vi "Images_Overlay_test.vi"() -> ()   [LabVIEW 2018]
uses:
  Common_Resources.lvlib
panel:
  out "error out":errorcluster
  out "Waveform Chart":dbl(graph)
  in  "Stop":bool
  in  "Image Display":T1(plugin-control)
  out "size(s)":i32[](array[numeric])
  in  "Overlay Object":path=path "D:/Users_Data/Dmitriy_T/Documents/Tracker/TestVI's/Overlay_Object.png"
  in  "Overlay Bgr":path=path "D:/Users_Data/Dmitriy_T/Documents/Tracker/TestVI's/Overlay_Bgr.png"
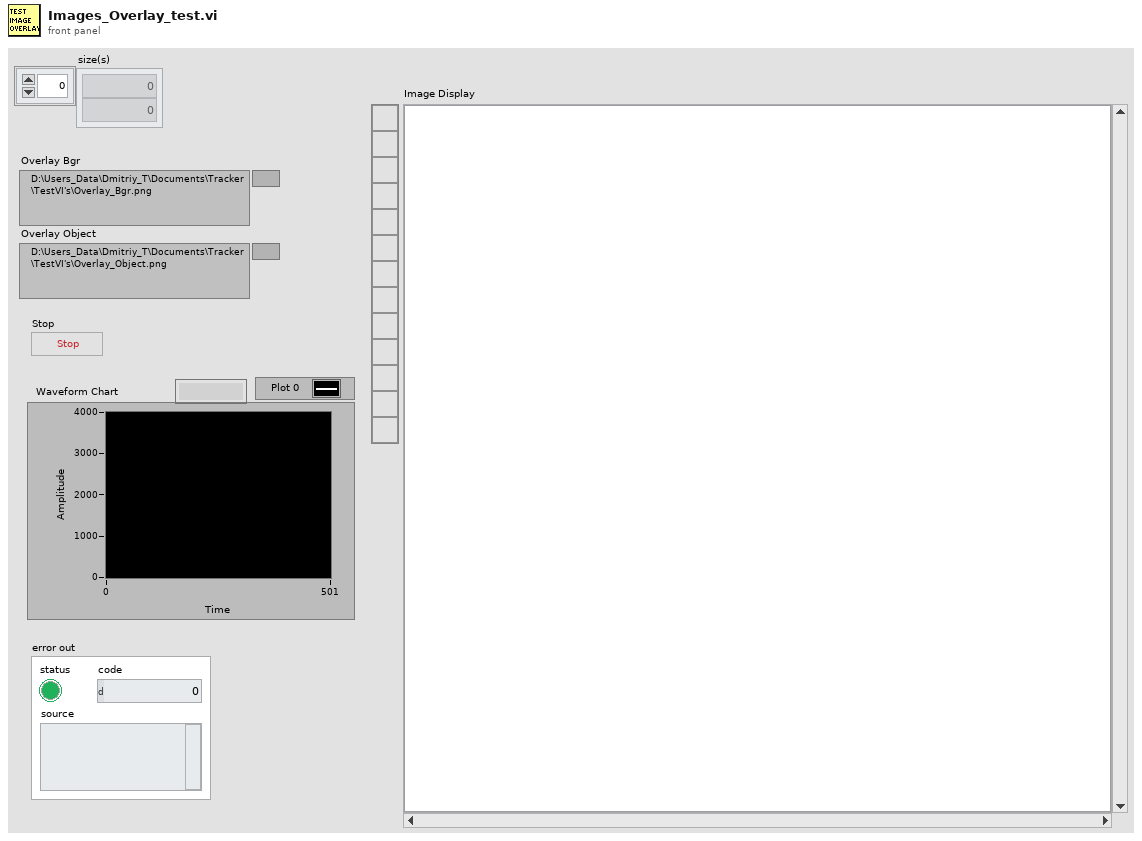
[diagram p1: front panel]
types:
  T1 = typedef "IMAQ Image.ctl" = refnum<image>
  T2 = typedef "Image Type" = u32
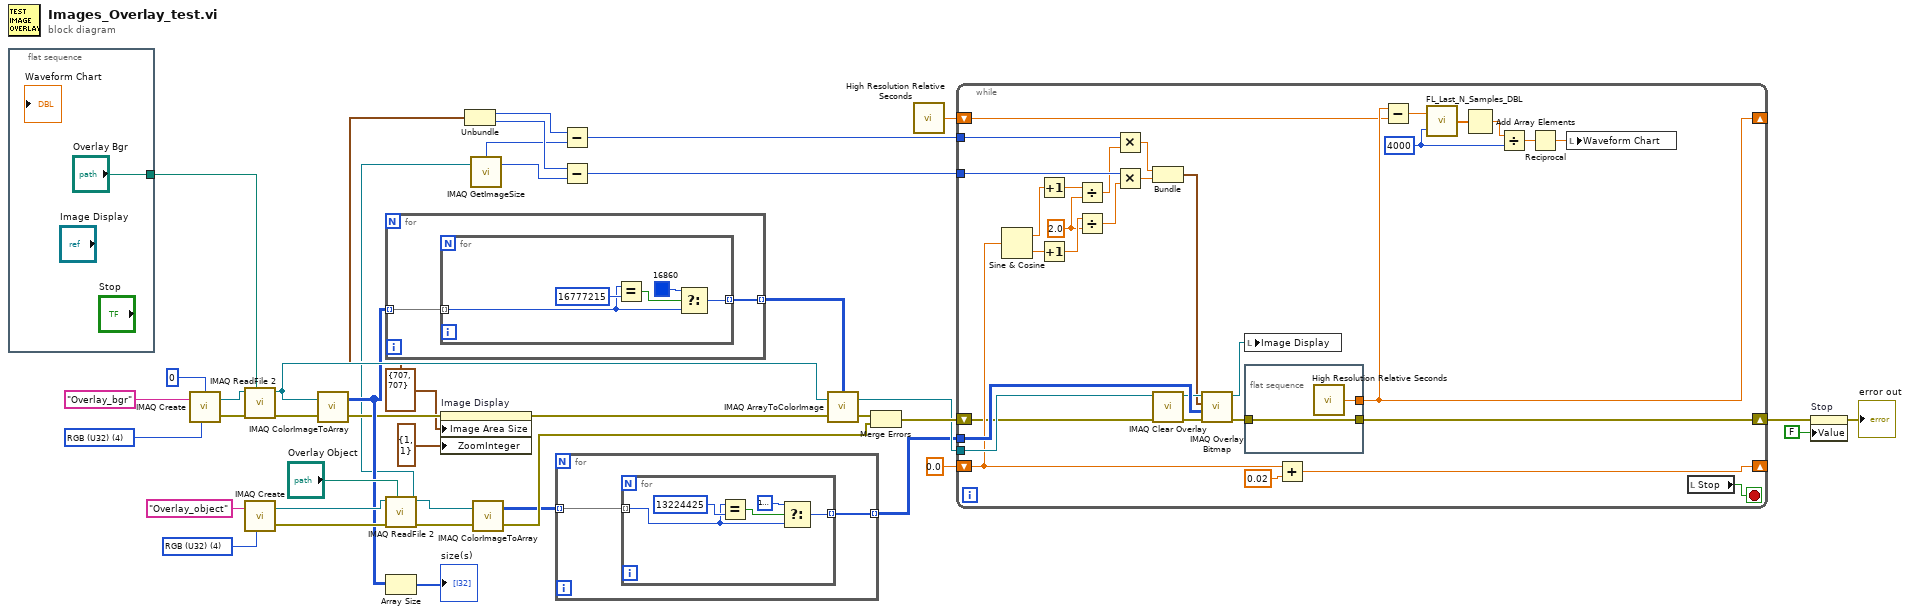
[diagram p0: block diagram]
diagram:
  w15 = cluster{"Width":u32, "Height":u32} {"Width"=707, "Height"=707} ("Image Area:Size:All Elements")
  w37 = T2 4 items=["Grayscale (U8)", "Grayscale (I16)", "Grayscale (SGL)", "Complex (CSG)", "RGB (U32)", "HSL (U32)", "RGB (U64)", "Grayscale (U16)"] ("Image Type")
  w38 = T2 4 items=["Grayscale (U8)", "Grayscale (I16)", "Grayscale (SGL)", "Complex (CSG)", "RGB (U32)", "HSL (U32)", "RGB (U64)", "Grayscale (U16)"] ("Image Type")
  n1 = flat-sequence {
    tunnel: ["Overlay Bgr"] -> w5
    frame #0 {
    }
  }
  n2 = call "IMAQ Create"("Border Size"=0, "Image Name"="Overlay_bgr", "Image Type"=w38) -> ("New Image"=w35:T1, "error out"=w34:errorcluster)  [unwired: 2 in]
  n3 = call "IMAQ ReadFile 2"("File Path"=w5, "error in (no error)"=w34, "Image"=w35) -> ("error out"=w26:errorcluster, "Image Out"=w23:T1)  [unwired: 4 in, 3 out]
  n4 = call "IMAQ Create"("Image Name"="Overlay_object", "Image Type"=w37) -> ("New Image"=w33:T1, "error out"=w32:errorcluster)  [unwired: 3 in]
  n5 = call "IMAQ ColorImageToArray"("Image"=w23, "error in (no error)"=w26) -> ("Image Pixels (U32)"=w22:u32[][], "error out"=w20:errorcluster)  [unwired: 2 in, 1 out]
  n6 = for {
    tunnel: w22 -> [w42] mode=indexing
    tunnel: [w41] -> w27 mode=indexing
    n7 = for {
      tunnel: w42 -> [w44] mode=indexing
      tunnel: [w46] -> w41 mode=indexing
      n8 = Equal?(x=w44, y=u32 16777215) -> (x = y?=w45:bool)
      n9 = Select(t=u32 16860, s=w45, f=w44) -> (s? t:f=w46:u32)
    }
  }
  n10 = call "IMAQ ReadFile 2"("File Path"="Overlay Object", "error in (no error)"=w32, "Image"=w33) -> ("error out"=w30:errorcluster, "Image Out"=w12:T1)  [unwired: 4 in, 3 out]
  n11 = Array Size(array=w22) -> (size(s)=→"size(s)":i32[])
  n12 = property on="Image Display" class="ImageControl"(error in=w20, "Image Area Size"=w15, "ZoomInteger"=cluster{"X":i32, "Y":i32} {"X"=1, "Y"=1} ("ZoomInteger:All Elements")) -> (error out=w19:errorcluster)  [unwired: 1 in, 1 out]
  n13 = Unbundle(w15) -> ("Width"=w14:u32, "Height"=w13:u32)
  n14 = call "IMAQ GetImageSize"("Image"=w12) -> ("Y Resolution"=w8:i32, "X Resolution"=w10:i32)  [unwired: 3 in, 1 out]
  n15 = call "IMAQ ColorImageToArray"("Image"=w12, "error in (no error)"=w30) -> ("Image Pixels (U32)"=w7:u32[][], "error out"=w29:errorcluster)  [unwired: 2 in, 1 out]
  n16 = for {
    tunnel: w7 -> [w49] mode=indexing
    tunnel: [w48] -> w6 mode=indexing
    n17 = for {
      tunnel: w49 -> [w51] mode=indexing
      tunnel: [w53] -> w48 mode=indexing
      n18 = Equal?(x=w51, y=u32 13224425) -> (x = y?=w52:bool)
      n19 = Select(t=u32 16777216, s=w52, f=w51) -> (s? t:f=w53:u32)
    }
  }
  n20 = Subtract(x=w14, y=w10) -> (x-y=w11:u32)
  n21 = Subtract(x=w13, y=w8) -> (x-y=w9:u32)
  n22 = call "IMAQ ArrayToColorImage"("Image Pixels (U32)"=w27, "Image"=w23, "error in (no error)"=w19) -> ("Image Out"=w24:T1, "error out"=w25:errorcluster)  [unwired: 2 in]
  n23 = Merge Errors(w25, w29) -> (w28:errorcluster)
  n24 = call <vilib>:"High Resolution Relative Seconds.vi"() -> ("relative seconds"=w1:dbl)
  n25 = while {
    tunnel: w6 -> [w86]
    tunnel: w24 -> [w85]
    shift-right: [w82] -> _
    shift-left: 0.0 -> [w84]
    tunnel: w11 -> [w81]
    tunnel: w9 -> [w79]
    shift-right: [w63] -> w4
    shift-left: w28 -> [w68]
    shift-right: [w62] -> _
    shift-left: w1 -> [w61]
    stop <- w66 stop-if-true
    w57 = 4000 ("BufferLengthSamples")
    w71 = 2.0 ("y")
    n26 = Sine & Cosine(0:w84) -> (1:w80:dbl, 2:w78:dbl)
    n27 = Increment(x=w80) -> (x+1=w75:dbl)
    n28 = Increment(x=w78) -> (x+1=w74:dbl)
    n29 = Divide(x=w75, y=w71) -> (x/y=w73:dbl)
    n30 = Divide(x=w74, y=w71) -> (x/y=w72:dbl)
    n31 = Multiply(x=w81, y=w73) -> (x*y=w76:dbl)
    n32 = Multiply(x=w79, y=w72) -> (x*y=w77:dbl)
    n33 = Bundle(w76, w77) -> (w65:cluster{dbl, dbl})  [unwired: 1 in]
    n34 = call "IMAQ Clear Overlay"("error in (no error)"=w68, "Image"=w85) -> ("error out"=w67:errorcluster, "Image Out"=w69:T1)  [unwired: 8 in]
    n35 = call "IMAQ Overlay Bitmap"("error in (no error)"=w67, "Bitmap"=w86, "Top Left Point"=w65, "Image"=w69) -> ("error out"=w64:errorcluster, "Image Out"=w70:T1)  [unwired: 6 in]
    n36 = local write "Image Display"(w70) -> ()
    n37 = flat-sequence {
      tunnel: w64 -> [w88]
      tunnel: [w88] -> w63
      tunnel: [w87] -> w62
      frame #0 {
        n38 = call <vilib>:"High Resolution Relative Seconds.vi"() -> ("relative seconds"=w87:dbl)
      }
    }
    n39 = Add(x=w84, y=0.02) -> (x+y=w82:dbl)
    n40 = Subtract(x=w62, y=w61) -> (x-y=w60:dbl)
    n41 = call "FL_Last_N_Samples_DBL.vi"("BufferLengthSamples"=w57, "Input sample"=w60) -> ("Output Array"=w59:dbl[])
    n42 = Add Array Elements(numeric array=w59) -> (sum=w58:dbl)
    n43 = Divide(x=w58, y=w57) -> (x/y=w56:dbl)
    n44 = Reciprocal(x=w56) -> (1/x=w55:dbl)
    n45 = local write "Waveform Chart"(w55) -> ()
    n46 = local read "Stop"() -> (w66:bool)
  }
  n47 = property on="Stop" class="Bool (strict)"(error in=w4, "Value"=FALSE ("Stop")) -> (error out=→"error out":errorcluster)  [unwired: 1 in, 1 out]
